vi "Destroy.vi"(8 "Error In":errorcluster, 11 "Object in":refnum<class "WebView.JSONEditor.lvclass">) -> (0 "Error Out":errorcluster)   [LabVIEW 2024, in "WebView.JSONEditor.lvclass"]
uses:
  WebView.JSONEditor.lvclass
  WebView_class/WebView.lvclass
  WebView.JSONEditor.lvclass/WebView.JSONEditor.ctl
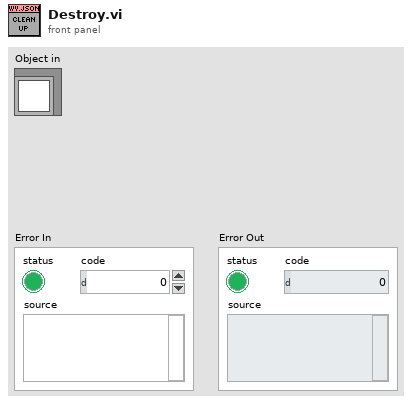
[diagram p1: front panel]
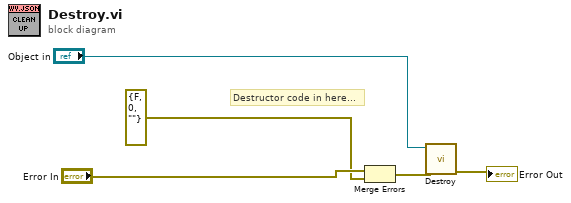
[diagram p0: block diagram]
diagram:
  # "Destructor code in here..."
  n1 = Merge Errors("Error In", errorcluster {"status"=FALSE, "code"=0, "source"=""} ("error in (no error)")) -> (w3:errorcluster)
  n2 = call-parent "Destroy.vi"("Error In"=w3, "WebView"="Object in") -> ("Error Out"=→"Error Out":errorcluster)  [unwired: 9 in]
